vi "DSF.Simulation.Custom Device.Create.vi"(8 "error in (no error)":errorcluster, 10 "Channel Count":u32, 11 "Simulated VeriStand Custom Device in":refnum<class "Simulated VeriStand Custom Device.lvclass">) -> (0 "error out":errorcluster, 3 "Simulated VeriStand Custom Device out":refnum<class "Simulated VeriStand Custom Device.lvclass">)   [LabVIEW 2016, in "Simulated VeriStand Custom Device.lvclass"]
uses:
  Simulated VeriStand Custom Device.lvclass
  Simulated VeriStand Custom Device.lvclass/Simulated VeriStand Custom Device.ctl
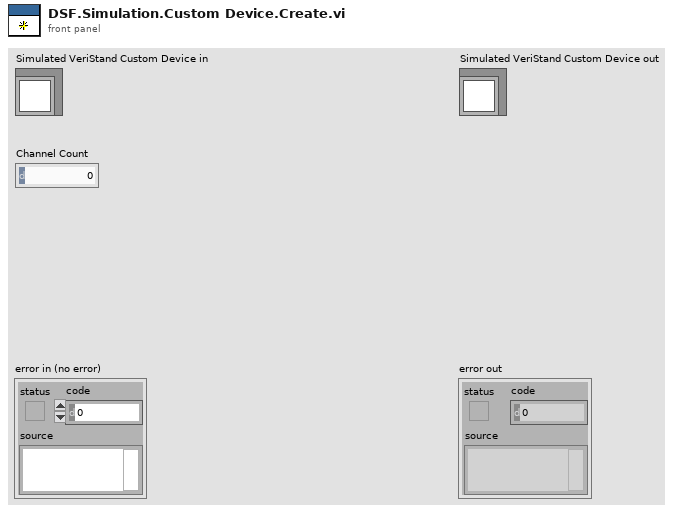
[diagram p1: front panel]
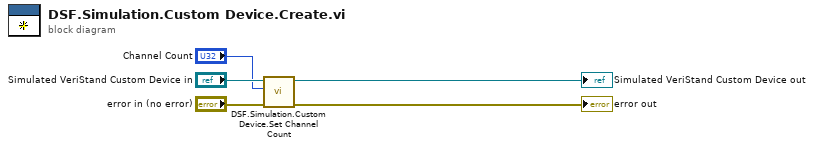
[diagram p0: block diagram]
diagram:
  n1 = call "DSF.Simulation.Custom Device.Set Channel Count.vi"("error in (no error)"="error in (no error)", "Channel Count"="Channel Count", "Simulated VeriStand Custom Device in"="Simulated VeriStand Custom Device in") -> ("error out"=→"error out":errorcluster, "Simulated VeriStand Custom Device out"=→"Simulated VeriStand Custom Device out":refnum<class "Simulated VeriStand Custom Device.lvclass">)  [unwired: 7 in]
